vi "Array Indexing.vi"(10 "Index":dbl, 11 "Array":dbl[](array[numeric]) caption="Array2") -> (3 "Result":dbl(knob) scale=0.0..10.0)   [LabVIEW 2024]
doc: "This VI selects an item from an array located at the given index."
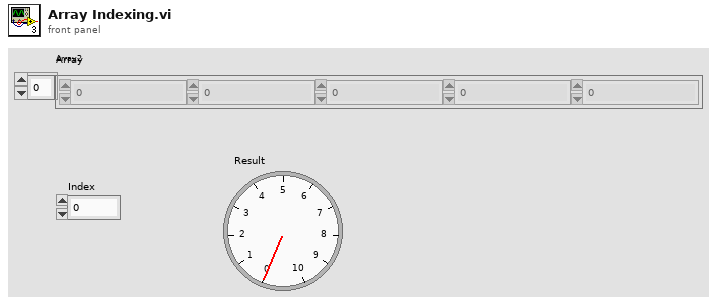
[diagram p1: front panel]
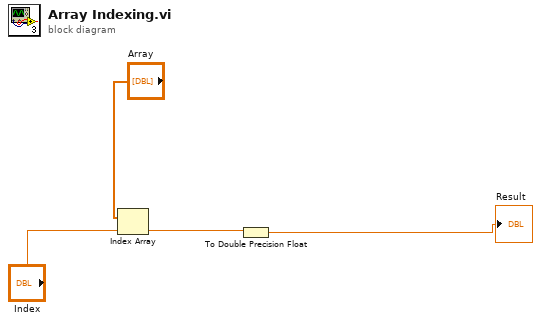
[diagram p0: block diagram]
diagram:
  n1 = Index Array(array="Array", index="Index") -> (element=w2:dbl)
  n2 = To Double Precision Float(number=w2) -> (double precision float=→"Result":dbl)
